vi "build.relative.vi"(10 "Time Unit":T1(ring), 11 "Time Series Name":string) -> (3 "ts.relative out":refnum<class "ts.relative.lvclass">)   [LabVIEW 2018, in "ts.relative.lvclass"]
uses:
  ts.relative.lvclass
  C:/code/labview-client/lv_src/timestampMetadata/timestampMetadata.lvclass
  timestampMetadata/timestampMetadata.lvclass/timestampMetadata.ctl
  ts.relative.lvclass/ts.relative.ctl
  timestampMetadata/seriesName.set.vi
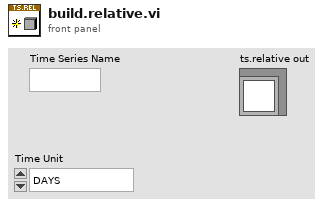
[diagram p1: front panel]
types:
  T1 = enum16{"DAYS", "HOURS", "MINUTES", "SECONDS", "MILLISECONDS", "MICROSECONDS", "NANOSECONDS", "PICOSECONDS"}
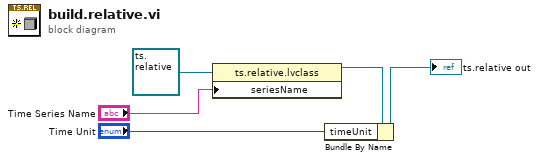
[diagram p0: block diagram]
diagram:
  n1 = property class="ts.relative.lvclass"(reference=refnum<class "ts.relative.lvclass"> refnum, "seriesName"="Time Series Name") -> (reference out=w2:refnum<class "ts.relative.lvclass">)  [unwired: 1 in, 1 out]
  n2 = Bundle By Name(cluster=w2, "timeUnit"="Time Unit") -> (→"ts.relative out":refnum<class "ts.relative.lvclass">)
